vi "setStatus.vi"(8 "error in (no error)":errorcluster, 10 "Status":T1, 11 "DAQmx in":refnum<class "DAQmx.lvclass">) -> (0 "error out":errorcluster, 3 "DAQmx out":refnum<class "DAQmx.lvclass">)   [LabVIEW 2019, in "DAQmx.lvclass"]
uses:
  DAQmx.lvclass
  typedefs/DAQmx.Status--enum.ctl
  DAQmx.lvclass/DAQmx.ctl
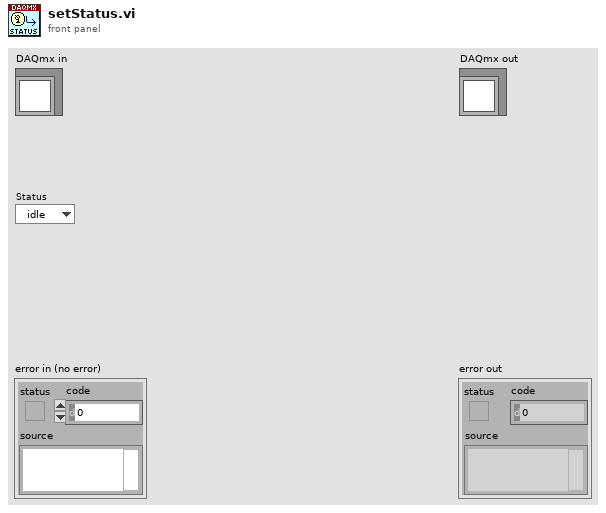
[diagram p1: front panel]
types:
  T1 = typedef "DAQmx.lvclass/DAQmx.Status--enum.ctl" = enum16{"idle", "calibrating", "configuring", "creating", "created", "starting", "started", "stopping", "stopped", "clearing", "error"}
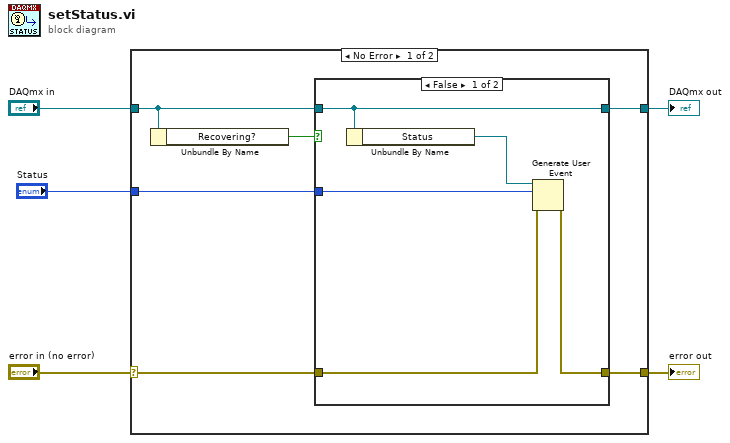
[diagram p0: block diagram]
diagram:
  n1 = case shown="No Error" "error in (no error)" {
    selector: "error in (no error)" -> [w11 w20]
    tunnel: [w10 w20] -> w4
    tunnel: [w6 w19] -> w2
    tunnel: "DAQmx in" -> [w8 w19]
    tunnel: "Status" -> [w9 _]
    frame No Error {
      n2 = Unbundle By Name(w8) -> ("Recovering?"=w7:bool)
      n3 = case shown="False" w7 {
        tunnel: w11 -> [w15 w17]
        tunnel: [w14 w17] -> w10
        tunnel: w9 -> [w13 _]
        tunnel: w8 -> [w12 w18]
        tunnel: [w12 w18] -> w6
        frame False {
          n4 = Unbundle By Name(w12) -> ("Status"=w16:refnum<user-event>)
          n5 = Generate User Event(user event=w16, event data cluster=w13, error in=w15) -> (error out=w14:errorcluster)  [unwired: 1 in, 1 out]
        }
        frame True {
        }
      }
    }
    frame Error {
    }
  }
  "error out" <- w4
  "DAQmx out" <- w2
